vi "exercicio5_boolean.vi"() -> ()   [LabVIEW 2018]
panel:
  out "x .and. y?":bool
  in  "Boolean 14":bool
  in  "Boolean 13":bool
  in  "Boolean 12":bool
  in  "Boolean 11":bool
  out "x .or. y?":bool
  in  "Boolean 10":bool
  in  "Boolean 9":bool
  in  "Boolean 8":bool
  out "result 2":bool
  in  "Boolean 7":bool
  in  "Boolean 6":bool
  in  "Boolean 5":bool
  out "result":bool
  in  "Boolean 4":bool
  in  "Boolean 3":bool
  in  "Boolean 2":bool
  in  "Boolean":bool
  # "Exercício 3"
  # "Exercício 1"
  # "Exercício 4"
  # "Exercício 2"
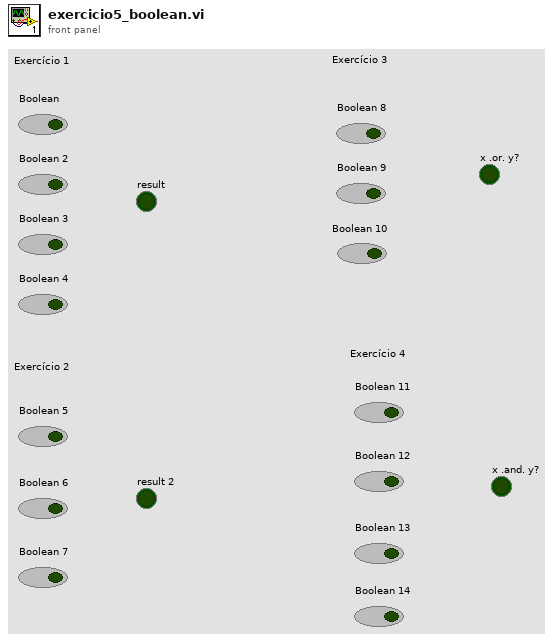
[diagram p1: front panel]
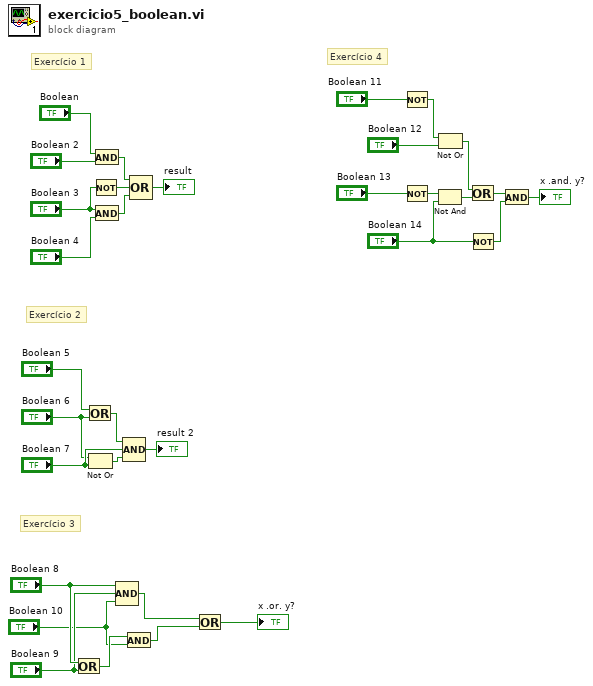
[diagram p0: block diagram]
diagram:
  # "Exercício 4"
  # "Exercício 3"
  # "Exercício 2"
  # "Exercício 1"
  n1 = Or(x="Boolean 8", y="Boolean 9") -> (x .or. y?=w16:bool)
  n2 = Or(x="Boolean 5", y="Boolean 6") -> (x .or. y?=w20:bool)
  n3 = Not Or(1:"Boolean 7", 2:"Boolean 6") -> (0:w21:bool)
  n4 = Not(x="Boolean 3") -> (.not. x?=w31:bool)
  n5 = And(x="Boolean", y="Boolean 2") -> (x .and. y?=w32:bool)
  n6 = And(x="Boolean 3", y="Boolean 4") -> (x .and. y?=w30:bool)
  n7 = Compound Arithmetic op=AND("Boolean 8", "Boolean 9", "Boolean 10") -> (w14:bool)
  n8 = Compound Arithmetic op=AND(w20, "Boolean 7", w21) -> (→"result 2":bool)
  n9 = And(x=w16, y="Boolean 10") -> (x .and. y?=w12:bool)
  n10 = Compound Arithmetic op=OR(w32, w31, w30) -> (→"result":bool)
  n11 = Or(x=w14, y=w12) -> (x .or. y?=→"x .or. y?":bool)
  n12 = Not(x="Boolean 11") -> (.not. x?=w11:bool)
  n13 = Not(x="Boolean 13") -> (.not. x?=w6:bool)
  n14 = Not Or(1:"Boolean 12", 2:w11) -> (0:w8:bool)
  n15 = Not And(1:"Boolean 14", 2:w6) -> (0:w5:bool)
  n16 = Or(x=w8, y=w5) -> (x .or. y?=w3:bool)
  n17 = Not(x="Boolean 14") -> (.not. x?=w2:bool)
  n18 = And(x=w3, y=w2) -> (x .and. y?=→"x .and. y?":bool)
